vi "_TEST_Get Excel Values.vi"() -> ()   [LabVIEW 2017, in "excel_configuration.lvlib"]
uses:
  excel_configuration.lvlib
  GetXL_CellValues_2D_Dbl.vi
panel:
  out "size(s)":i32
  out "data":dbl[][](array[numeric])
  in  "Sheet":i32=1
  out "error out":errorcluster
  in  "End":cluster{"Column":i32, "Row":i32}={"Column"=1, "Row"=2}
  in  "Start":cluster{"Column":i32, "Row":i32}={"Column"=1, "Row"=1}
  in  "path":path
  # "1. Specify the path to the workbook.\n2. Specify the specific sheet. If you use a string\n    control instead of a numeric control you can\n    specify the sheet by its name.\n3. Specify the start and end positions in terms\n    of rows and columns (unit-indexed).\n4. If you want to read the data in as a string,\n    or if you want to read in only a single cell,\n    go to the block diagram and change the\n    polymorphic instance of the GetXL_Values\n    VI to the appropriate parameter. Create\n    an indicator for the new instance.\n5. Press run to extract the data from the Excel\n    workbook as specified."
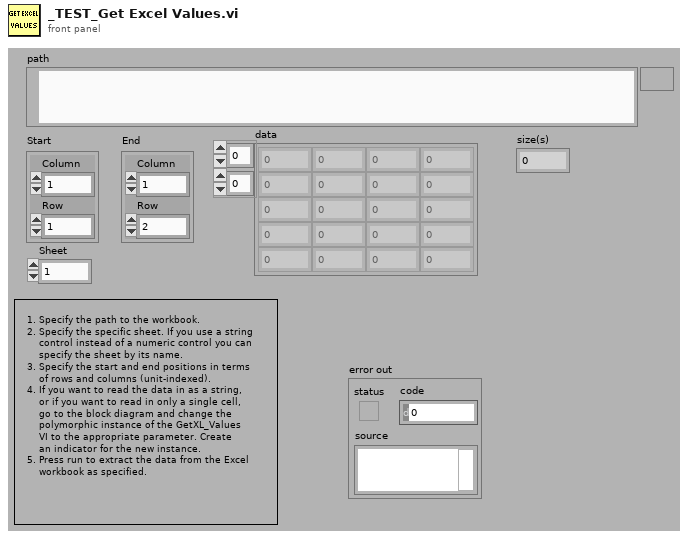
[diagram p1: front panel]
types:
  T1 = cluster{"Excel._Application":refnum<k7>, "Workbooks":refnum<k7>}
  T2 = cluster{"Excel._Application":refnum<k7>, "Workbooks":refnum<k7>, "Open":refnum<k7>}
  T3 = cluster{"Excel._Application":refnum<k7>, "Workbooks":refnum<k7>, "Open":refnum<k7>, "Worksheets":refnum<k7>, "Excel._Worksheet":refnum<k7>}
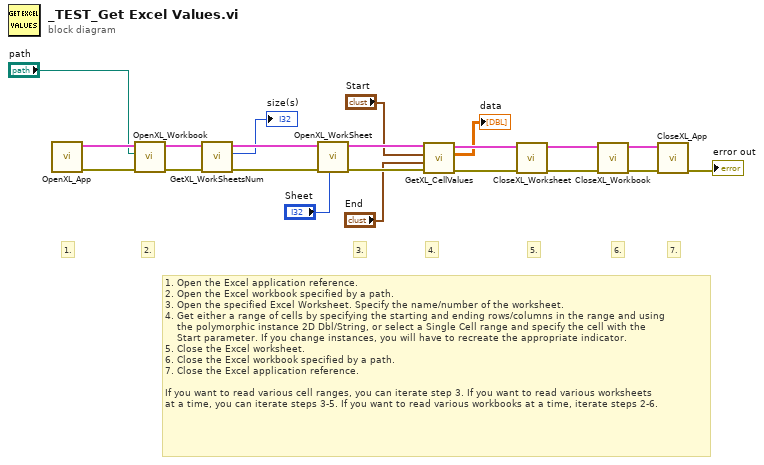
[diagram p0: block diagram]
diagram:
  # "7."
  # "4."
  # "1. Open the Excel application reference.\n2. Open the Excel workbook specified by a path.\n3. Open the specified Excel Worksheet. Specify the name/number of the worksheet.\n4. Get either a range of cells by specifying the starting and ending rows/columns in the range and using\n    the polymorphic instance 2D Dbl/String, or select a Single Cell range and specify the cell with the \n    Start parameter. If you change instances, you will have to recreate the appropriate indicator.\n5. Close the Excel worksheet.\n6. Close the Excel workbook specified by a path.\n7. Close the Excel application reference.\n\nIf you want to read various cell ranges, you can iterate step 3. If you want to read various worksheets\nat a time, you can iterate steps 3-5. If you want to read various workbooks at a time, iterate steps 2-6."
  # "6."
  # "5."
  # "3."
  # "2."
  # "1."
  n1 = call "OpenXL_App.vi"() -> ("error out"=w13:errorcluster, "Refnum Cluster"=w14:T1)  [unwired: 10 in]
  n2 = call "OpenXL_Workbook.vi"("error in"=w13, "path"="path", "Refnum Cluster In"=w14) -> ("error out"=w3:errorcluster, "Refnum Cluster Out"=w5:T2)  [unwired: 7 in]
  n3 = call "GetXL_WorkSheetsNum.vi"("error in (no error)"=w3, "Refnum Cluster In"=w5) -> ("error out"=w2:errorcluster, "size(s)"=→"size(s)":i32, "Refnum Cluster In"=w4:T2)  [unwired: 7 in]
  n4 = call "OpenXL_WorkSheet.vi"("Sheet"="Sheet", "error in (no error)"=w2, "Refnum Cluster In"=w4) -> ("error out"=w20:errorcluster, "Refnum Cluster Out"=w21:T3)  [unwired: 7 in]
  n5 = call-poly "GetXL_CellValues.vi"("error in"=w20, "End"="End", "Start"="Start", "Refnum Cluster In"=w21) -> ("error out"=w10:errorcluster, "data"=→"data":dbl[][], "Refnum Cluster Out"=w11:T3)  [unwired: 5 in]
  n6 = call "CloseXL_Worksheet.vi"("error in (no error)"=w10, "Refnum Cluster In"=w11) -> ("error out"=w8:errorcluster, "Refnum Cluster Out"=w9:T2)  [unwired: 8 in]
  n7 = call "CloseXL_Workbook.vi"("error in (no error)"=w8, "Refnum Cluster In"=w9) -> ("error out"=w18:errorcluster, "Refnum Cluster Out"=w19:T1)  [unwired: 8 in]
  n8 = call "CloseXL_App.vi"("error in (no error)"=w18, "Refnum Cluster In"=w19) -> ("error out"=→"error out":errorcluster)  [unwired: 9 in]
